vi "Setflex_ray_comm.vi"(8 "error in (no error)":errorcluster, 10 "Set_Val":T1, 11 "OneOfTemplate in":refnum<class "nixnet_grpc_ReadStateValue_value.lvclass">) -> (0 "error out":errorcluster, 3 "OneOfTemplate out":refnum<class "nixnet_grpc_ReadStateValue_value.lvclass">)   [LabVIEW 2019, in "grpc-xnet_client.lvlib" / "nixnet_grpc_ReadStateValue_value.lvclass"]
uses:
  nixnet_grpc_ReadStateValue_value.lvclass
  nixnet_grpc_FlexRayCommResponse.ctl
  nixnet_grpc_FlexRayPocState.ctl
  nixnet_grpc_ReadStateValue_value.lvclass/nixnet_grpc_ReadStateValue_value.ctl
  grpc-xnet_client.lvlib
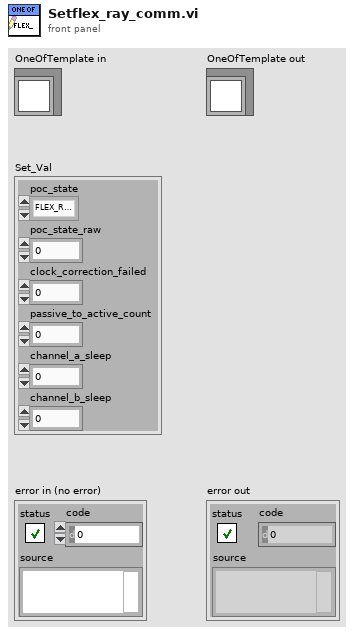
[diagram p1: front panel]
types:
  T1 = typedef "grpc-xnet_client.lvlib/nixnet_grpc_FlexRayCommResponse.ctl" = cluster{"poc_state":T2, "poc_state_raw":u32, "clock_correction_failed":u32, "passive_to_active_count":u32, "channel_a_sleep":u32, "channel_b_sleep":u32}
  T2 = typedef "grpc-xnet_client.lvlib/nixnet_grpc_FlexRayPocState.ctl" = enum32{"FLEX_RAY_POC_STATE_DEFAULT_CONFIG", "FLEX_RAY_POC_STATE_READY", "FLEX_RAY_POC_STATE_NORMAL_ACTIVE", "FLEX_RAY_POC_STATE_NORMAL_PASSIVE", "FLEX_RAY_POC_STATE_HALT", "FLEX_RAY_POC_STATE_MONITOR", "FLEX_RAY_POC_STATE_CONFIG"}
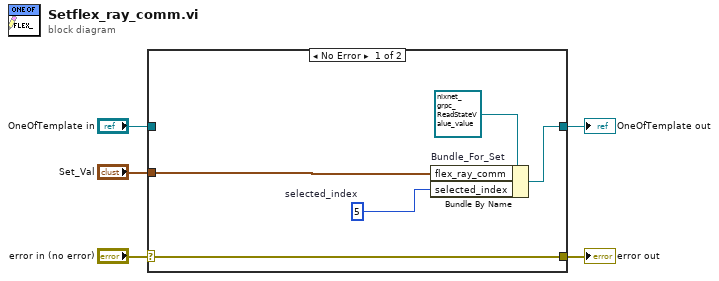
[diagram p0: block diagram]
diagram:
  n1 = case shown="No Error" "error in (no error)" {
    selector: "error in (no error)" -> [w10 w11]
    tunnel: [w10 w11] -> w4
    tunnel: [w9 w12] -> w2
    tunnel: "OneOfTemplate in" -> [_ w12]
    tunnel: "Set_Val" -> [w8 _]
    frame No Error {
      w7 = 5  # selected_index
      n2 = Bundle By Name "Bundle_For_Set"(cluster=refnum<class "nixnet_grpc_ReadStateValue_value.lvclass"> refnum ("OneOfTemplate in"), "flex_ray_comm"=w8, "selected_index"=w7) -> (w9:refnum<class "nixnet_grpc_ReadStateValue_value.lvclass">)
    }
    frame Error {
    }
  }
  "error out" <- w4
  "OneOfTemplate out" <- w2
